vi "oa_Compute D and beta Kaiser Filter Parameters.vi"(11 "A stop":dbl) -> (2 "beta":dbl, 3 "D":dbl)   [LabVIEW 2017, in "SoundVib_RefDataProcess.lvlib"]
uses:
  <vilib>/addons/Sound and Vibration/Order Analysis/Referece Data Processing/SoundVib_RefDataProcess.lvlib
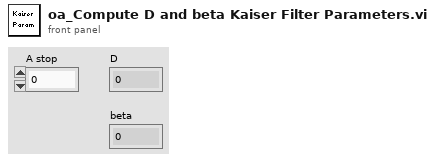
[diagram p1: front panel]
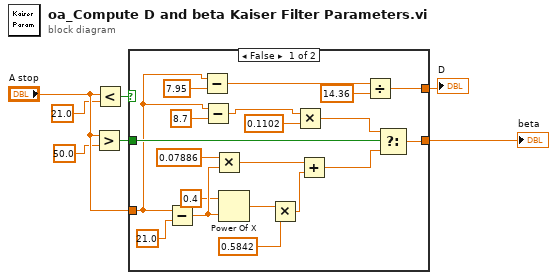
[diagram p0: block diagram]
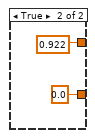
[diagram p2: hidden frame]
diagram:
  n1 = Greater?(x="A stop", y=50.0) -> (0:w4:bool)
  n2 = Less?(x="A stop", y=21.0) -> (x < y?=w5:bool)
  n3 = case shown="False" w5 {
    tunnel: "A stop" -> [w12 _]
    tunnel: [w20 0.0 ("t")] -> w3
    tunnel: w4 -> [w19 _]
    tunnel: [w14 0.922 ("t")] -> w6
    frame False {
      n4 = Subtract(x=w12, y=21.0) -> (x-y=w18:dbl)
      n5 = Subtract(x=w12, y=7.95) -> (x-y=w16:dbl)
      n6 = Subtract(x=w12, y=8.7) -> (x-y=w10:dbl)
      n7 = Multiply(x=0.07886, y=w18) -> (x*y=w22:dbl)
      n8 = Power Of X(1:w18, 2:0.4 ("x")) -> (0:w26:dbl)
      n9 = Multiply(x=w26, y=0.5842) -> (x*y=w23:dbl)
      n10 = Multiply(x=w10, y=0.1102) -> (x*y=w8:dbl)
      n11 = Add(x=w22, y=w23) -> (x+y=w21:dbl)
      n12 = Divide(x=w16, y=14.36) -> (x/y=w14:dbl)
      n13 = Select(t=w8, s=w19, f=w21) -> (s? t:f=w20:dbl)
    }
    frame True {
    }
  }
  "D" <- w6
  "beta" <- w3
